vi "Set Command Line.vi"(8 "error in (no error)":errorcluster, 9 "arguments":string[](array[string]), 10 "path":path, 11 "subprocess in":refnum<class "Buffered Subprocess.lvclass">) -> (0 "error out":errorcluster, 3 "subprocess out":refnum<class "Buffered Subprocess.lvclass">)   [LabVIEW 2020, in "NI_Subprocess.lvlib" / "Buffered Subprocess.lvclass"]
uses:
  <vilib>/Subprocess/Buffered Subprocess/Buffered Subprocess.lvclass
  <vilib>/Subprocess/Buffered Subprocess/Buffered Subprocess.lvclass/Buffered Subprocess.ctl
  <vilib>/Subprocess/Subprocess/Subprocess.lvclass
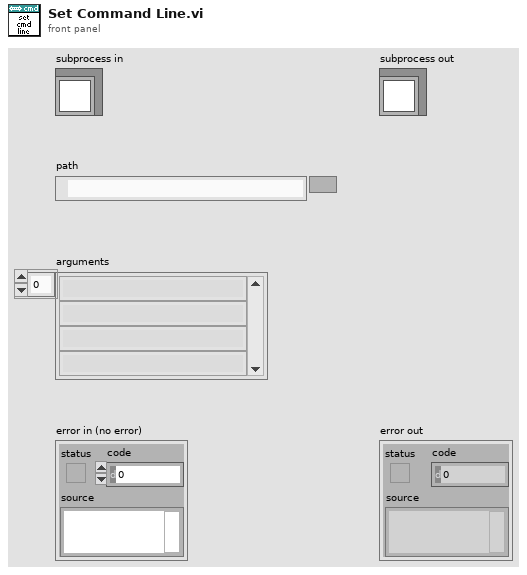
[diagram p1: front panel]
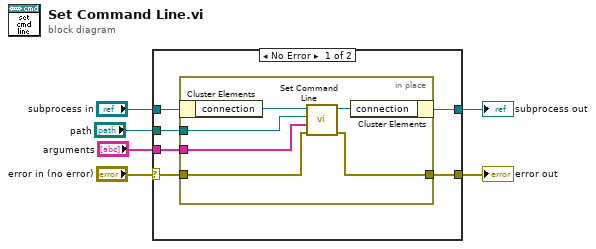
[diagram p0: block diagram]
diagram:
  n1 = case shown="No Error" "error in (no error)" {
    selector: "error in (no error)" -> [w11 w20]
    tunnel: [w9 w20] -> w5
    tunnel: [w10 w19] -> w3
    tunnel: "subprocess in" -> [w12 w19]
    tunnel: "path" -> [w8 _]
    tunnel: "arguments" -> [w7 _]
    frame No Error {
      n2 = in-place {
        in-place-border: w11 -> [w16]
        in-place-border: [w15] -> w9
        in-place-border: w8 -> [w14]
        in-place-border: w7 -> [w13]
        n3 = in-place-cluster #1(w12) -> ("connection"=w18:refnum<class "Subprocess.lvclass">)
        n4 = call <vilib>:"Set Command Line.vi"("error in (no error)"=w16, "arguments"=w13, "path"=w14, "subprocess in"=w18) -> ("error out"=w15:errorcluster, "subprocess out"=w17:refnum<class "Subprocess.lvclass">)  [unwired: 6 in]
        n5 = in-place-cluster #1("connection"=w17) -> (w10:refnum<class "Buffered Subprocess.lvclass">)
      }
    }
    frame Error {
    }
  }
  "error out" <- w5
  "subprocess out" <- w3
